vi "TestEvaluateTriggerCondition.vi"() -> ()   [LabVIEW 2017]
uses:
  <vilib>/addons/InsightCM/Devices/Shared/Common/Trigger/controls/TriggerCondition.ctl
  <vilib>/addons/InsightCM/MessageBus/Base/controls/Condition.ctl
  <vilib>/addons/PointValueMap/subVIs/Point_Write_double.vi
  <vilib>/addons/InsightCM/Utilities/GlobalConfiguration/GlobalConfiguration.lvlib
  <vilib>/addons/PointValueMap/PointValueMap.lvlib
  <vilib>/addons/InsightCM/Devices/Shared/Common/Trigger/Trigger.lvlib
panel:
  in  "Expression":string
  out "trigger":bool
  out "error out":errorcluster
  in  "Value":dbl=5.0
  in  "BlockSizeSeconds":dbl=1.0
  in  "Conditions":T1[](array[typedef])=[{"Condition"={"Source"="", "Type"="", "Operator"="", "CompareTo"="", "DwellSeconds"=0.0}, "LatchValue"="", "LatchTime"=timestamp(0 s since 1904-01-01)}]
  in  "Next":bool
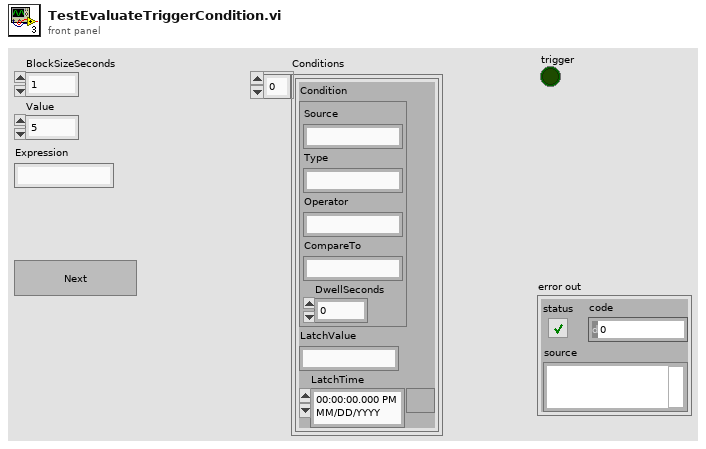
[diagram p1: front panel]
types:
  T1 = typedef "Trigger.lvlib/TriggerCondition.ctl" = cluster{"Condition":T2, "LatchValue":string, "LatchTime":timestamp}
  T2 = typedef "Condition.ctl" = cluster{"Source":string, "Type":string, "Operator":string, "CompareTo":string, "DwellSeconds":dbl}
  T3 = typedef "PointValueMap.lvlib/PointMap.ctl" = refnum<data-value>
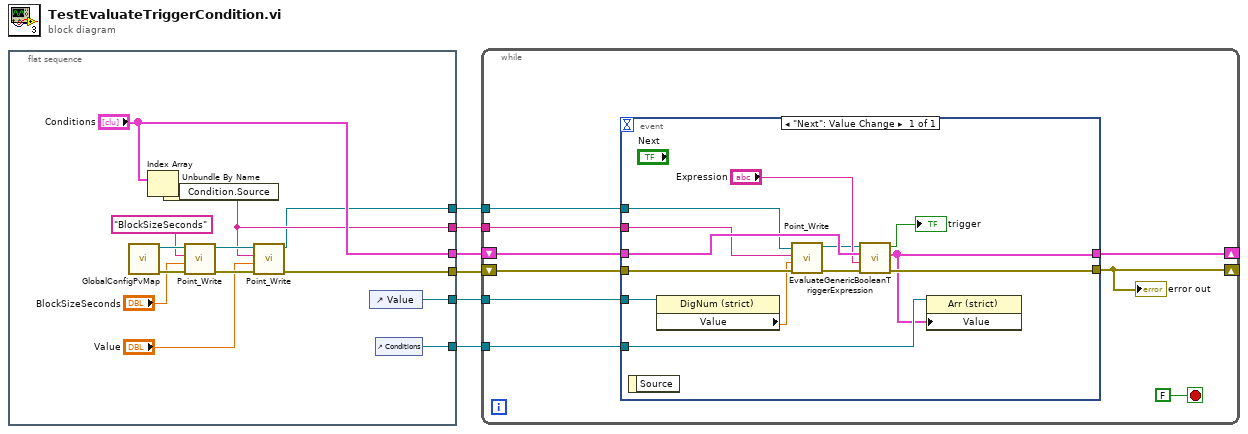
[diagram p0: block diagram]
diagram:
  n1 = flat-sequence {
    tunnel: [w11] -> w6
    tunnel: [w7] -> w5
    tunnel: ["Conditions"] -> w4
    tunnel: [w12] -> w3
    tunnel: [w9] -> w2
    tunnel: [w8] -> w1
    frame #0 {
      n2 = call <vilib>:"GlobalConfigPvMap.vi"() -> ("error out"=w19:errorcluster, "global configuration map"=w20:T3)  [unwired: 10 in]
      n3 = Index Array(array="Conditions") -> (element=w18:T1)  [unwired: 1 in]
      n4 = Unbundle By Name(w18) -> ("Condition.Source"=w8:string)
      n5 = call-poly <vilib>:"Point_Write.vi"("Error In"=w19, "Value"="BlockSizeSeconds", "Tag"="BlockSizeSeconds", "Map"=w20) -> ("Error Out"=w14:errorcluster, "Map Out"=w15:T3)  [unwired: 6 in]
      n6 = call-poly <vilib>:"Point_Write.vi"("Error In"=w14, "Value"="Value", "Tag"=w8, "Map"=w15) -> ("Error Out"=w11:errorcluster, "Map Out"=w7:T3)  [unwired: 6 in]
      n7 = control-ref of="Value"() -> (w12:refnum<vi>)
      n8 = control-ref of="Conditions"() -> (w9:refnum<vi>)
    }
  }
  n9 = while {
    shift-right: [w28] -> _
    shift-left: w6 -> [w27]
    tunnel: w5 -> [w26]
    shift-right: [w25] -> _
    shift-left: w4 -> [w24]
    tunnel: w3 -> [w23]
    tunnel: w2 -> [w22]
    tunnel: w1 -> [w21]
    stop <- FALSE stop-if-true
    n10 = event shown="[0] \"Next\": Value Change" {
      selector: _ -> [_]
      dyn-events: _ -> [_]
      timeout: _ -> [_]
      tunnel: [w42] -> w28
      tunnel: w27 -> [w37]
      tunnel: w26 -> [w36]
      tunnel: [w39] -> w25
      tunnel: w24 -> [w41]
      tunnel: w23 -> [w38]
      tunnel: w22 -> [w40]
      tunnel: w21 -> [w33]
      event "Next": Value Change {
        n11 = event-data() -> ()  [unwired: 1 in, 1 out]
        n12 = property class="DigNum (strict)"(reference=w38) -> ("Value"=w34:dbl)  [unwired: 1 in, 2 out]
        n13 = call-poly <vilib>:"Point_Write.vi"("Error In"=w37, "Value"=w34, "Tag"=w33, "Map"=w36) -> ("Error Out"=w35:errorcluster, "Map Out"=w30:T3)  [unwired: 6 in]
        n14 = call <vilib>:"EvaluateGenericBooleanTriggerExpression.vi"("error in (no error)"=w35, "expression"="Expression", "all conditions"=w41, "map"=w30) -> ("error out"=w42:errorcluster, "all conditions out"=w39:T1[], "trigger"=→"trigger":bool)  [unwired: 4 in, 1 out]
        n15 = property class="Arr (strict)"(reference=w40, "Value"=w39) -> ()  [unwired: 1 in, 2 out]
      }
    }
    "error out" <- w28
  }
